vi "GetDataFormat.vi"(8 "Error In":errorcluster, 11 "Keithley 6482 In":refnum<visa-resource-name>) -> (0 "Error Out":errorcluster, 2 "Data Format":T1, 3 "Keithley 6482 Out":refnum<visa-resource-name>)   [LabVIEW 2012, in "Keithley-6482.lvlib"]
uses:
  Keithley-6482.lvlib
  Controls/DataFormat.ctl
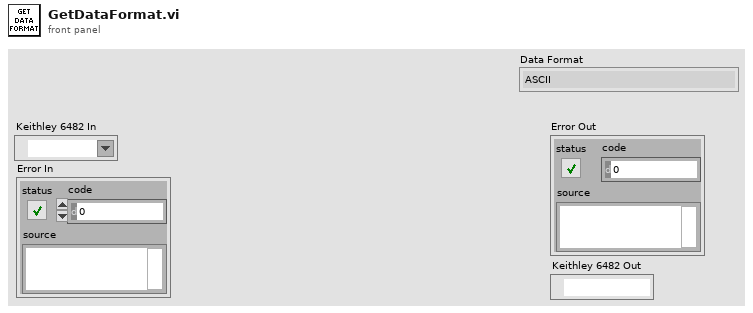
[diagram p1: front panel]
types:
  T1 = typedef "Keithley-6482.lvlib/DataFormat.ctl" = enum16{"ASCII", "Real", "32", "Sreal"}
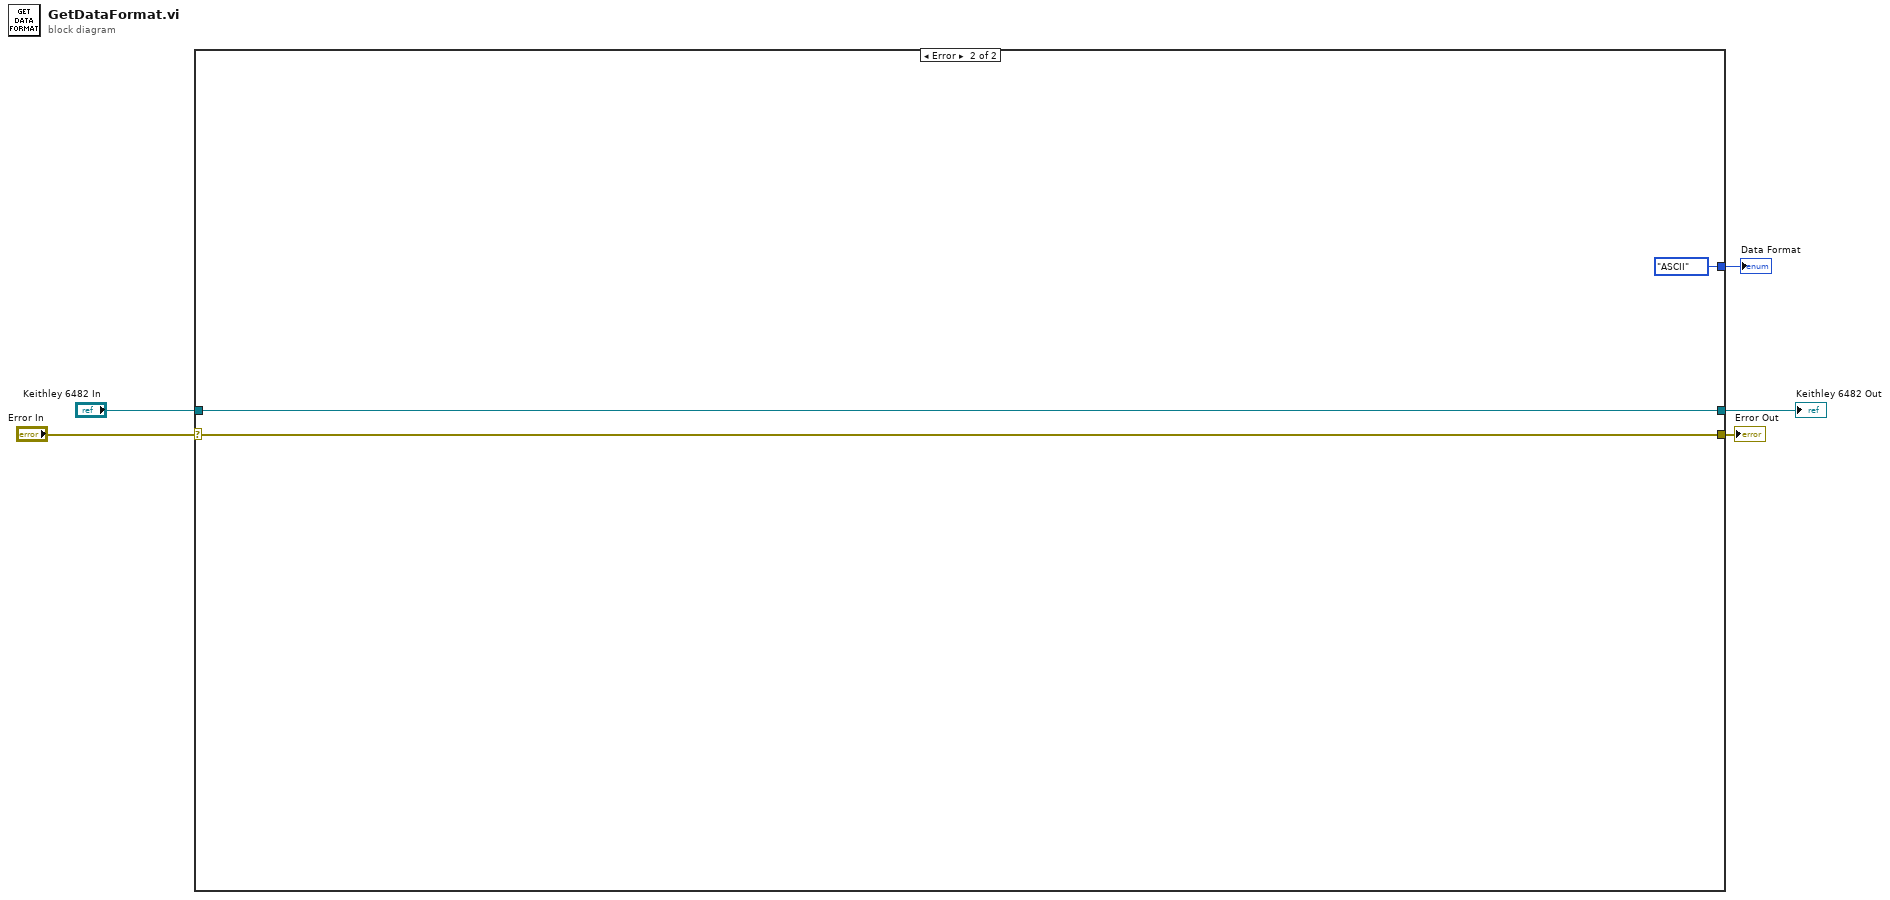
[diagram p0: block diagram]
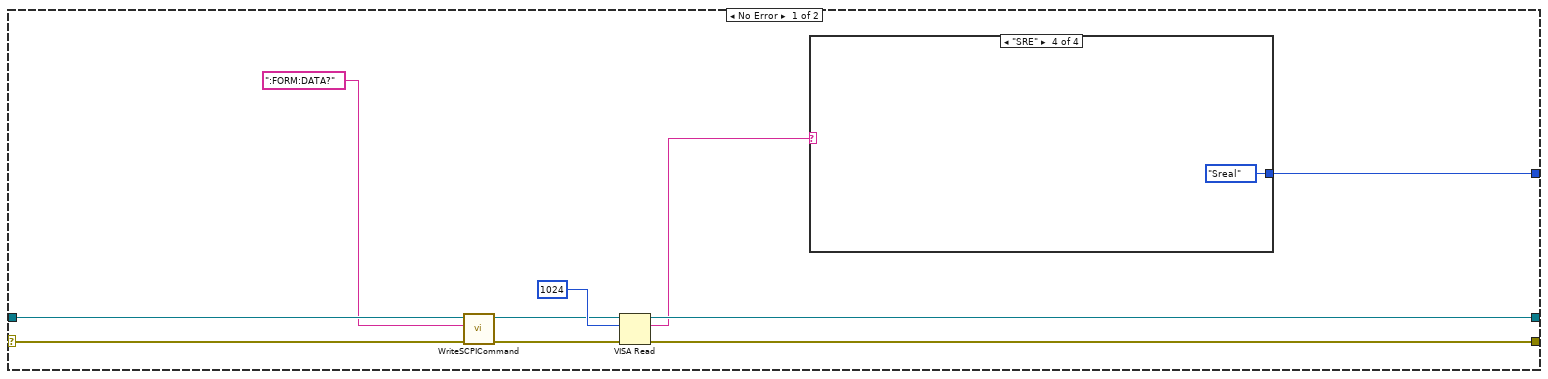
[diagram p2: hidden frame]
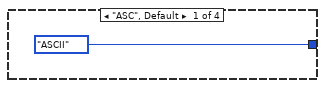
[diagram p3: hidden frame]
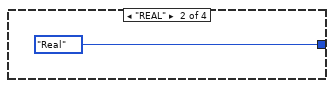
[diagram p4: hidden frame]
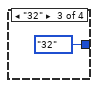
[diagram p5: hidden frame]
diagram:
  n1 = case shown="Error" "Error In" {
    selector: "Error In" -> [w10 w21]
    tunnel: "Keithley 6482 In" -> [w9 w22]
    tunnel: [w15 w21] -> w3
    tunnel: [w14 w22] -> w2
    tunnel: [w6 DataFormat."ASCII" ("Data Format")] -> w1
    frame No Error {
      n2 = call "WriteSCPICommand.vi"("Error In"=w10, "SCPI Command"=":FORM:DATA?", "Keithley 6482 In"=w9) -> ("Error Out"=w11:errorcluster, "Keithley 6482 Out"=w12:refnum<visa-resource-name>)  [unwired: 7 in]
      n3 = VISA Read(VISA resource name=w12, byte count=u32 1024, error in (no error)=w11) -> (VISA resource name out=w14:refnum<visa-resource-name>, read buffer=w7:string, error out=w15:errorcluster)  [unwired: 1 out]
      n4 = case shown="\"SRE\"" w7 {
        tunnel: [DataFormat."ASCII" ("Data Format") DataFormat."Real" ("Data Format") DataFormat."32" ("Data Format") DataFormat."Sreal" ("Data Format")] -> w6
        frame "ASC", Default {
        }
        frame "REAL" {
        }
        frame "32" {
        }
        frame "SRE" {
        }
      }
    }
    frame Error {
    }
  }
  "Error Out" <- w3
  "Keithley 6482 Out" <- w2
  "Data Format" <- w1
